vi "Gergberg.vi"() -> ()   [LabVIEW 2012, in "LightPipes.lvlib"]
uses:
  LightPipes.lvlib
panel:
  in  "Forward Distance":dbl(slide)=-2.439454888092385e-19 step=0.0001 scale=-0.02..0.02
  in  "stop":bool
  out "Distance":dbl=-2.439454888092385e-19
  out "Iteration":i32=49
  out "Original Far Field":T1(plugin-control)
  out "Original Mid Field":T1(plugin-control)
  out "error out":errorcluster
  in  "error in (no error)":errorcluster
  out "Far Field":T1(plugin-control)
  out "MF Phase":T1(plugin-control)
  out "Target Intensity\n RMS Error":dbl(graph)=169.26733826023644
  out "FF Phase":T1(plugin-control)
  out "Mid Field":T1(plugin-control)
  in  "Image Size":i32=300
  in  "lambda":dbl=1.054e-06
  in  "forward distance":dbl=0.02
  in  "size_grid":dbl=0.001776
  in  "Number of Iteration":i32=50
  in  "Far Field":path=path "E:/data4/FF Centered.png"
  in  "Mid Field":path=path "E:/data4/MF Centered.png"
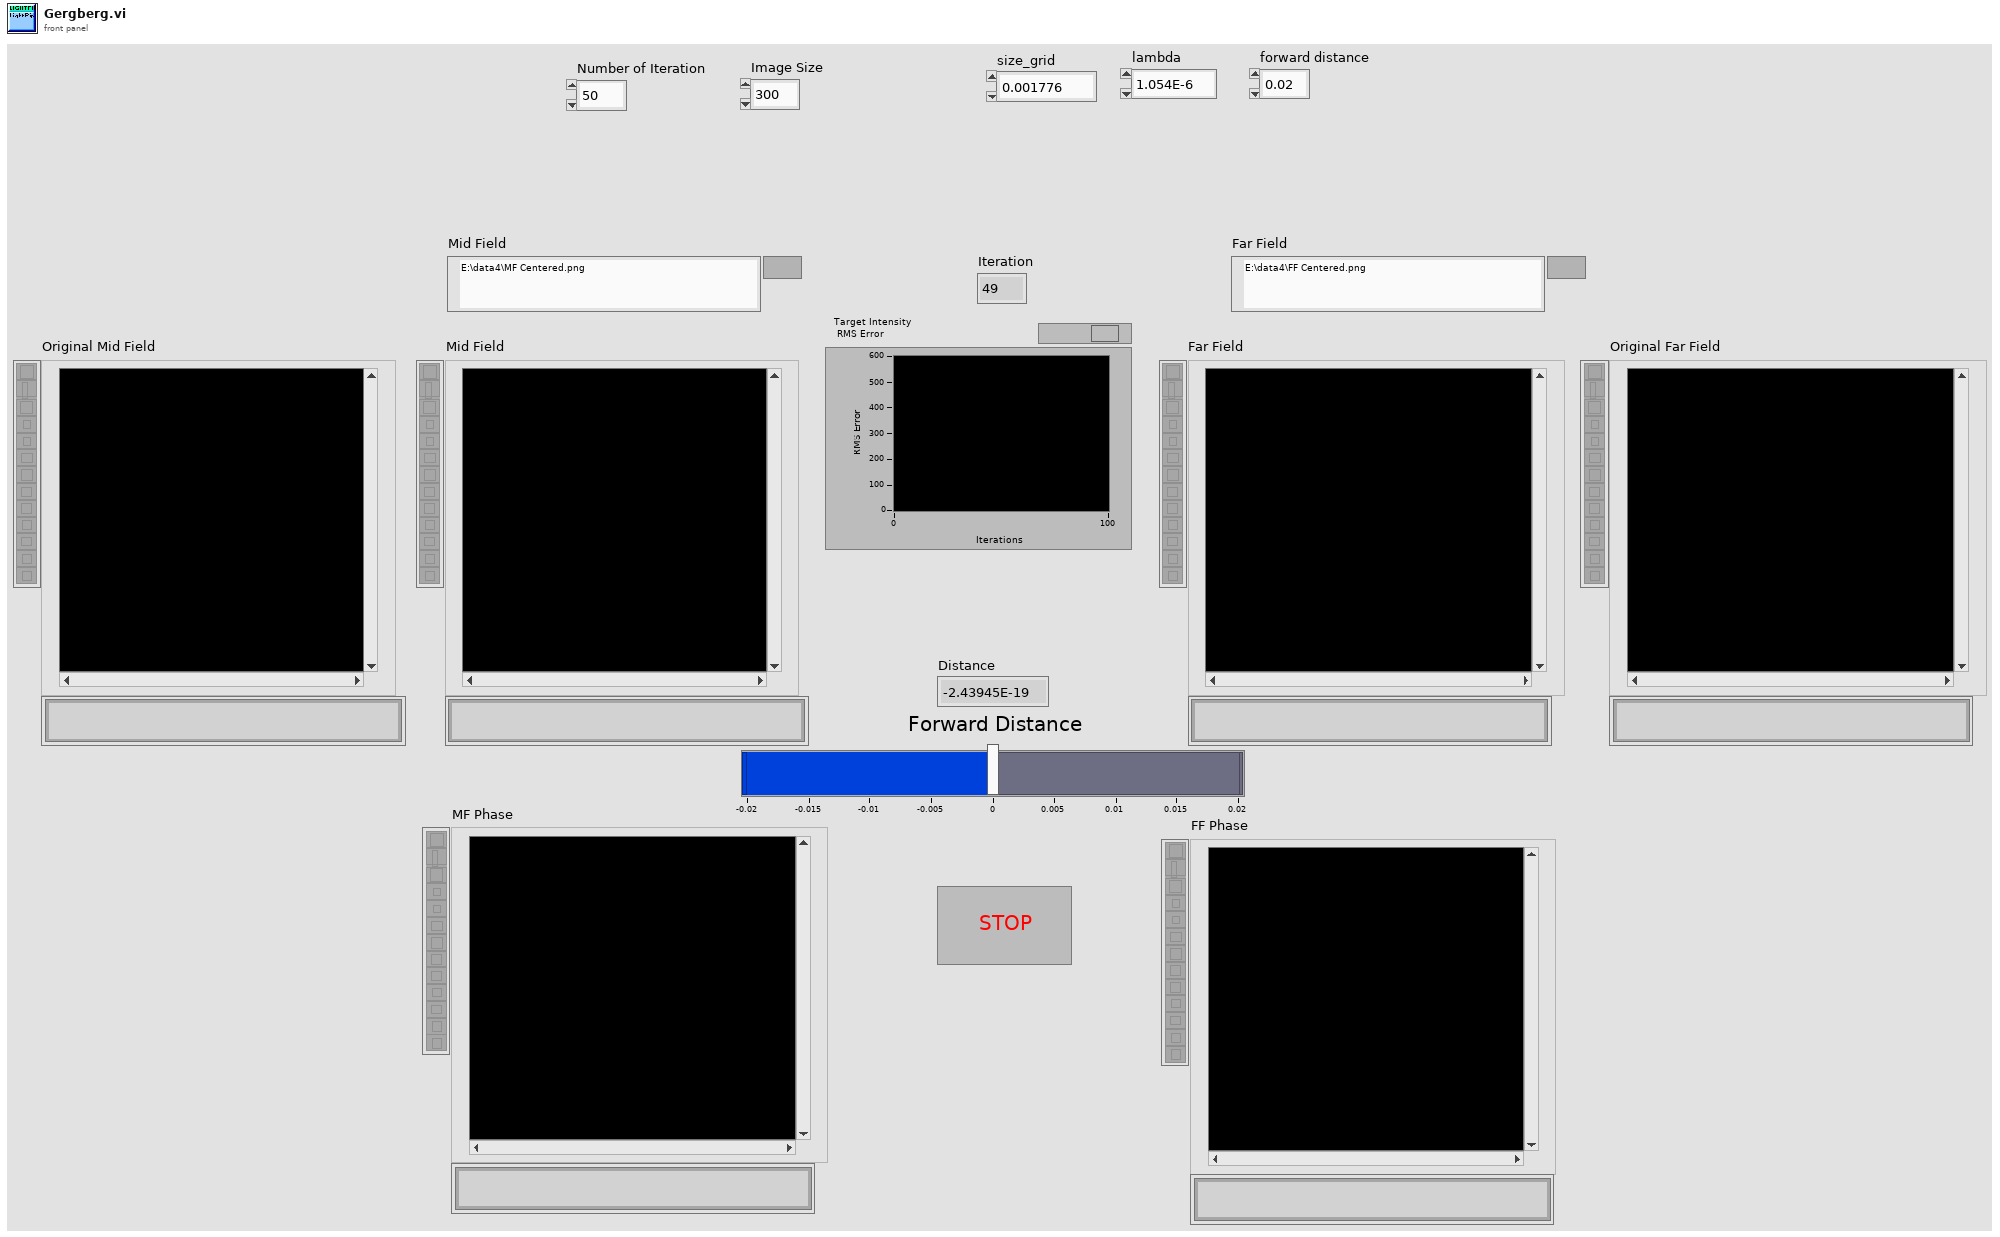
[diagram p1: front panel]
types:
  T1 = typedef "IMAQ Image.ctl" = refnum<image>
  T2 = typedef "Image Type" = u32
  T3 = cluster{"n_grid":i32, "@dummy control@":i8, "@dummy control@":i8, "@dummy control@":i8, "@dummy control@":i8, "size":dbl, "lambda":dbl, "int1":i32, "int2":i32, "int3":i32, "@dummy control@":i8, "@dummy control@":i8, "@dummy control@":i8, "@dummy control@":i8, "double1":dbl, "double2":dbl, "double3":dbl, "real":u32, "imaginary":u32}
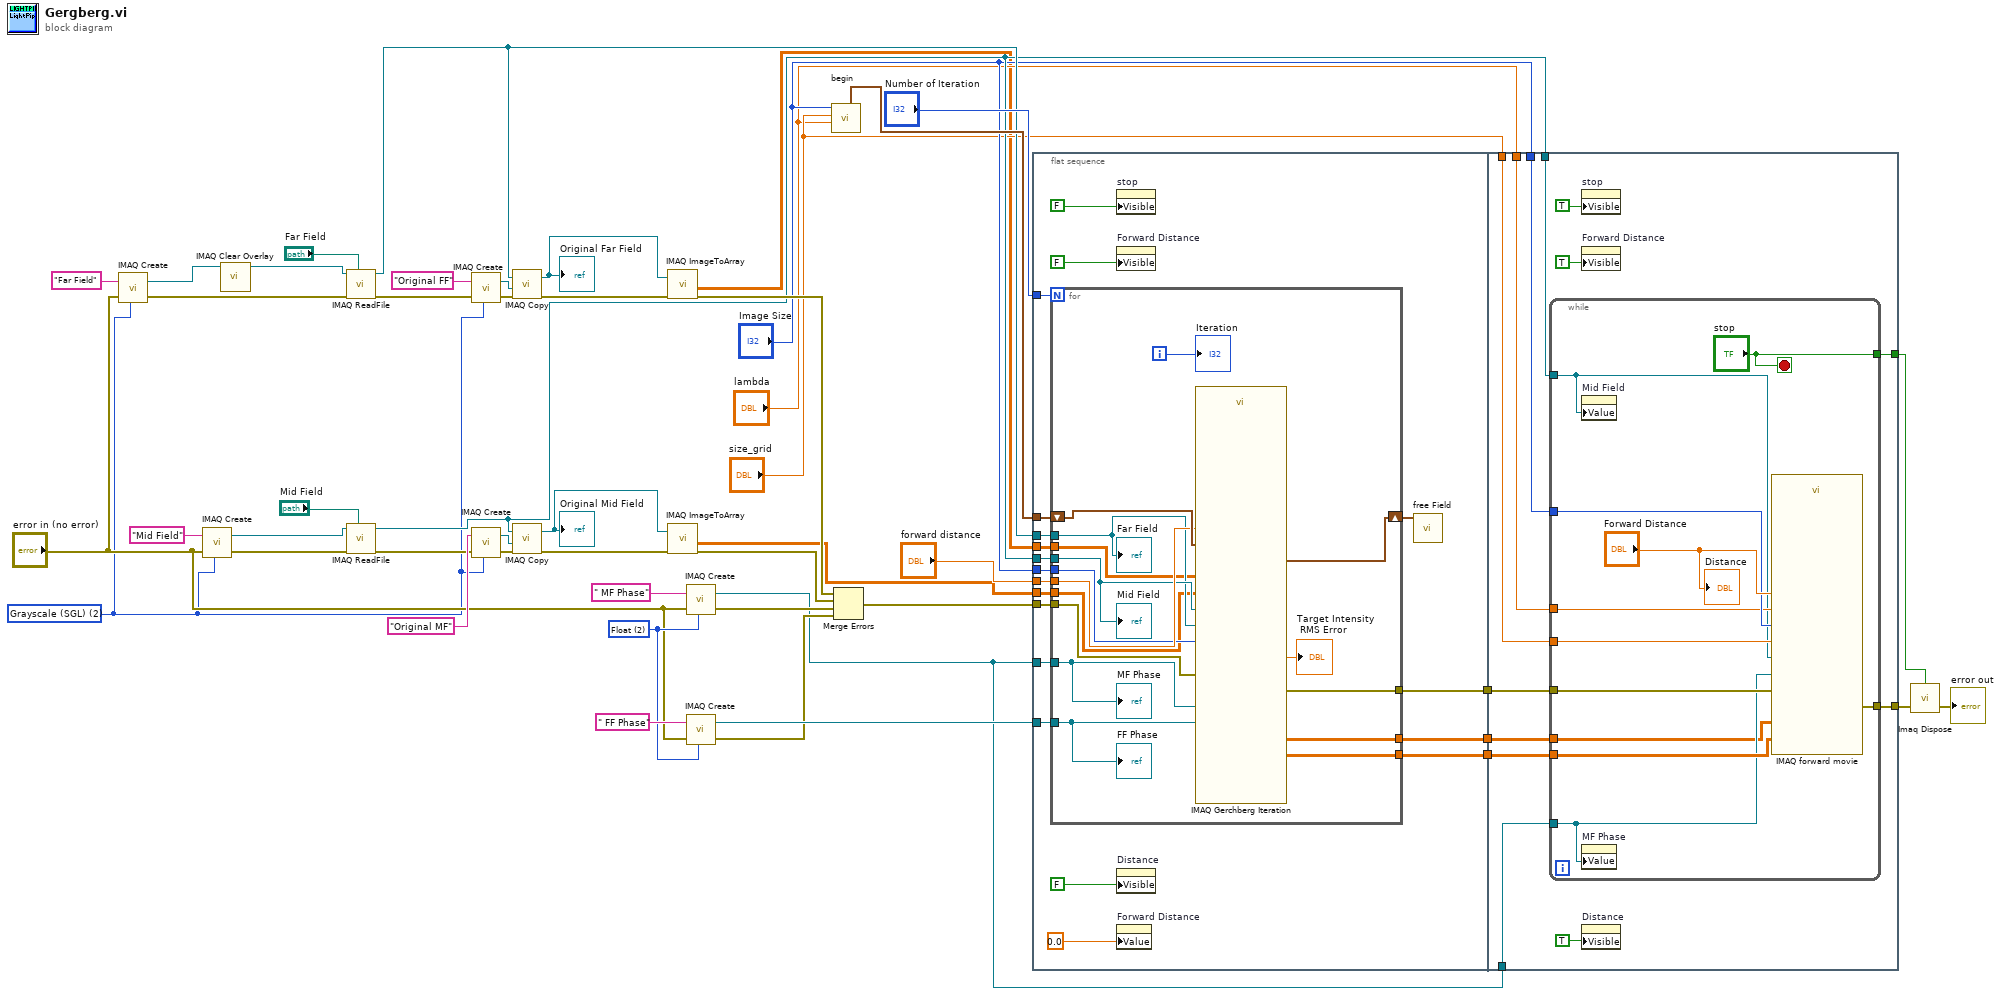
[diagram p0: block diagram]
diagram:
  w3 = T2 2 items=["Grayscale (U8)", "Grayscale (I16)", "Grayscale (SGL)", "Complex (CSG)", "RGB (U32)", "HSL (U32)", "RGB (U64)", "Grayscale (U16)"] ("Intensity Image Type")
  w42 = u32 2 items=["8 bits", "16 bits", "Float", "Complex", "RGB", "HSL"] ("Image Type")
  n1 = call "IMAQ Create"("Image Name"="Far Field", "Image Type"=w3, "error in (no error)"="error in (no error)") -> ("New Image"=w17:T1, "error out"=w29:errorcluster)  [unwired: 2 in]
  n2 = call "IMAQ Create"("Image Name"="Mid Field", "Image Type"=w3, "error in (no error)"="error in (no error)") -> ("New Image"=w43:T1, "error out"=w27:errorcluster)  [unwired: 2 in]
  n3 = call "IMAQ Clear Overlay"("Image"=w17) -> ("Image Out"=w16:T1)  [unwired: 9 in, 1 out]
  n4 = call "IMAQ ReadFile"("File Path"="Far Field", "error in (no error)"=w29, "Image"=w16) -> ("error out"=w28:errorcluster, "Image Out"=w30:T1)  [unwired: 2 in, 5 out]
  n5 = call "IMAQ ReadFile"("File Path"="Mid Field", "error in (no error)"=w27, "Image"=w43) -> ("error out"=w26:errorcluster, "Image Out"=w10:T1)  [unwired: 2 in, 5 out]
  n6 = call "IMAQ Create"("Image Name"="Original FF", "Image Type"=w3, "error in (no error)"=w28) -> ("New Image"=w38:T1, "error out"=w37:errorcluster)  [unwired: 2 in]
  n7 = call "IMAQ Create"("Image Name"="Original MF", "Image Type"=w3, "error in (no error)"=w26) -> ("New Image"=w41:T1, "error out"=w40:errorcluster)  [unwired: 2 in]
  n8 = call "IMAQ Copy"("error in (no error)"=w37, "Image Dst"=w38, "Image Src"=w30) -> ("error out"=w32:errorcluster, "Image Dst Out"=w18:T1)  [unwired: 3 in]
  "Original Far Field" <- w18
  n9 = call "IMAQ Copy"("error in (no error)"=w40, "Image Dst"=w41, "Image Src"=w10) -> ("error out"=w31:errorcluster, "Image Dst Out"=w19:T1)  [unwired: 3 in]
  "Original Mid Field" <- w19
  n10 = call "IMAQ ImageToArray"("error in (no error)"=w32, "Image"=w18) -> ("Image Pixels (Float)"=w2:sgl[][], "error out"=w25:errorcluster)  [unwired: 2 in, 3 out]
  n11 = call "IMAQ ImageToArray"("error in (no error)"=w31, "Image"=w19) -> ("Image Pixels (Float)"=w1:sgl[][], "error out"=w24:errorcluster)  [unwired: 2 in, 3 out]
  n12 = call "IMAQ Create"("Image Name"=" MF Phase", "Image Type"=w42, "error in (no error)"="error in (no error)") -> ("New Image"=w11:T1, "error out"=w21:errorcluster)  [unwired: 2 in]
  n13 = call "IMAQ Create"("Image Name"=" FF Phase", "Image Type"=w42, "error in (no error)"="error in (no error)") -> ("New Image"=w22:T1, "error out"=w20:errorcluster)  [unwired: 2 in]
  n14 = call "begin.vi"("lambda"="lambda", "size_grid"="size_grid", "n_grid"="Image Size") -> ("field out"=w34:T3)  [unwired: 8 in]
  n15 = Merge Errors(w25, w24, w21, w20) -> (w23:errorcluster)
  n16 = flat-sequence {
    tunnel: "Number of Iteration" -> [w68]
    tunnel: w34 -> [w67]
    tunnel: "forward distance" -> [w66]
    tunnel: w10 -> [w64]
    tunnel: w30 -> [w63]
    tunnel: w23 -> [w62]
    tunnel: "Image Size" -> [w61]
    tunnel: w22 -> [w60]
    tunnel: w11 -> [w59]
    tunnel: w1 -> [w52]
    tunnel: w2 -> [w58]
    tunnel: [w57] -> w14
    tunnel: [w51] -> w5
    tunnel: [w54] -> w4
    tunnel: w14 -> [w85]
    tunnel: [w96] -> w12
    tunnel: w11 -> [w88]
    tunnel: w10 -> [w89]
    tunnel: "Image Size" -> [w95]
    tunnel: "size_grid" -> [w94]
    tunnel: "lambda" -> [w93]
    tunnel: [w92] -> w6
    tunnel: w5 -> [w87]
    tunnel: w4 -> [w86]
    frame #0 {
      n17 = for {
        N: w68 -> [_]
        shift-right: [w83] -> w65
        shift-left: w67 -> [w84]
        tunnel: w66 -> [w82]
        tunnel: w52 -> [w70]
        tunnel: w58 -> [w71]
        tunnel: w64 -> [w77]
        tunnel: w63 -> [w76]
        tunnel: w62 -> [w81]
        tunnel: [w80] -> w57
        tunnel: w61 -> [w79]
        tunnel: w60 -> [w73]
        tunnel: w59 -> [w74]
        tunnel: [w72] -> w54
        tunnel: [w69] -> w51
        i -> [w78]
        n18 = call "IMAQ Gerchberg Iteration.vi"("field"=w84, "Original Source"=w70, "n_grid"=w79, "forward distance"=w82, "Original Target"=w71, "error in (no error)"=w81, "Source"=w77, "Target"=w76, "Source Phase"=w74, "Target Phase"=w73) -> ("Source Intensity"=w69:dbl[][], "Source Phase"=w72:dbl[][], "field out"=w83:T3, "Target Intensity\n RMS Error"=→"Target Intensity\n RMS Error":dbl, "error out"=w80:errorcluster)  [unwired: 3 in, 2 out]
        "Iteration" <- w78
        "Mid Field" <- w77
        "Far Field" <- w76
        "MF Phase" <- w74
        "FF Phase" <- w73
      }
      n19 = property on="stop" class="Bool"("Visible"=FALSE) -> ()  [unwired: 2 in, 2 out]
      n20 = property on="Forward Distance" class="Slide (strict)"("Visible"=FALSE) -> ()  [unwired: 2 in, 2 out]
      n21 = property on="Distance" class="DigNum (strict)"("Visible"=FALSE) -> ()  [unwired: 2 in, 2 out]
      n22 = property on="Forward Distance" class="Slide (strict)"("Value"=0.0 ("Forward Distance")) -> ()  [unwired: 2 in, 2 out]
      n23 = call "free Field.vi"("field"=w65) -> ()  [unwired: 10 in, 1 out]
    }
    frame #1 {
      n24 = while {
        tunnel: ["stop"] -> w96
        tunnel: w88 -> [w99]
        tunnel: w89 -> [w100]
        tunnel: w95 -> [w107]
        tunnel: w94 -> [w106]
        tunnel: w93 -> [w105]
        tunnel: [w102] -> w92
        tunnel: w85 -> [w103]
        tunnel: w87 -> [w98]
        tunnel: w86 -> [w101]
        stop <- "stop" stop-if-true
        n25 = property on="Mid Field" class="ImageControl"("Value"=w100) -> ()  [unwired: 2 in, 2 out]
        n26 = property on="MF Phase" class="ImageControl"("Value"=w99) -> ()  [unwired: 2 in, 2 out]
        n27 = call "IMAQ forward movie.vi"("Forwarded Phase"=w99, "n_grid"=w107, "Source Intensity"=w98, "Forwarded Intensity"=w100, "error in (no error)"=w103, "size_grid"=w106, "lambda"=w105, "Forward Distance"="Forward Distance", "Source Phase"=w101) -> ("error out"=w102:errorcluster)  [unwired: 6 in]
        "Distance" <- "Forward Distance"
      }
      n28 = property on="stop" class="Bool"("Visible"=TRUE) -> ()  [unwired: 2 in, 2 out]
      n29 = property on="Forward Distance" class="Slide (strict)"("Visible"=TRUE) -> ()  [unwired: 2 in, 2 out]
      n30 = property on="Distance" class="DigNum (strict)"("Visible"=TRUE) -> ()  [unwired: 2 in, 2 out]
    }
  }
  n31 = call "Imaq Dispose"("All Images? (No)"=w12, "error in (no error)"=w6) -> ("error out"=→"error out":errorcluster)  [unwired: 4 in]
